vi "Get UDP Reference.vi"(8 "error in (no error)":errorcluster, 11 "Assert Name":string) -> (0 "error out":errorcluster, 2 "UDP Reference":refnum<k16>)   [LabVIEW 2016, in "Assert API Components.lvlib" / "Log Assert Core.lvlib"]
uses:
  Log Assert Core.lvlib
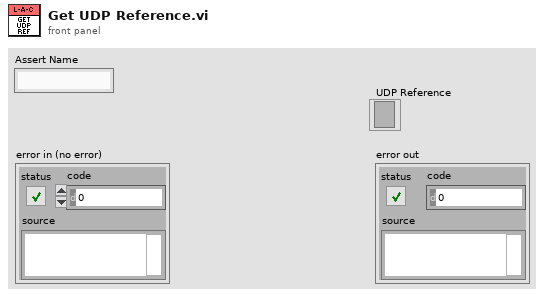
[diagram p1: front panel]
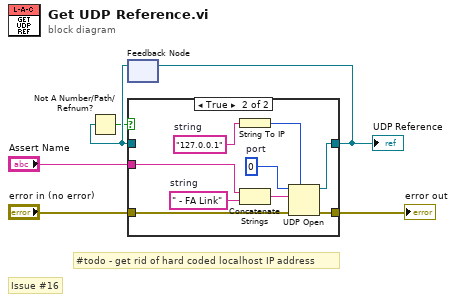
[diagram p0: block diagram]
diagram:
  # "Issue #16"
  # "#todo - get rid of hard coded localhost IP address"
  n1 = feedback #1() -> (w6:refnum<k16>)  [unwired: 1 in]
  n2 = Not A Number/Path/Refnum?(number/path/refnum=w6) -> (NaN/Path/Refnum?=w5:bool)
  n3 = case shown="True" w5 {
    tunnel: "error in (no error)" -> [w7 w17]
    tunnel: [w7 w16] -> w2
    tunnel: [w8 w14] -> w4
    tunnel: w6 -> [w8 _]
    tunnel: "Assert Name" -> [_ w13]
    frame False {
    }
    frame True {
      w10 = "127.0.0.1"  # string
      w12 = " - FA Link"  # string
      w15 = u16 0  # port
      n4 = String To IP(1:w10) -> (0:w9:u32)
      n5 = Concatenate Strings(w13, w12) -> (w11:string)
      n6 = UDP Open(7:w9, 8:w17, 10:w11, 11:w15) -> (port=w14:refnum<k16>, 0:w16:errorcluster)  [unwired: 1 in, 1 out]
    }
  }
  "error out" <- w2
  "UDP Reference" <- w4
  n7 = feedback-in #1(w4) -> ()
